vi "GetStringEnumTerminals.vi"(8 "error in (no error)":errorcluster, 9 "WireTerminal":refnum<vi>, 11 "Terms[]":refnum<vi>[](array[refnum])) -> (0 "error out":errorcluster, 3 "Array":refnum<vi>[](array[refnum]))   [LabVIEW 2020, in "Scripting.lvclass"]
uses:
  Scripting.lvclass
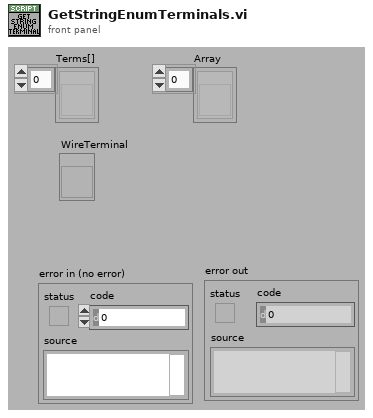
[diagram p1: front panel]
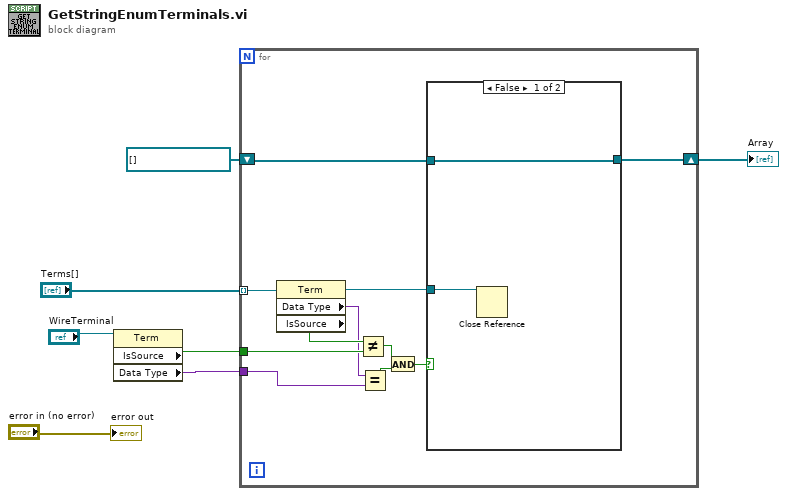
[diagram p0: block diagram]
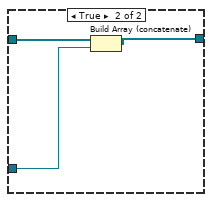
[diagram p2: hidden frame]
diagram:
  n1 = property class="Term"(reference="WireTerminal") -> ("IsSource"=w3:bool, "Data Type"=w2:variant)  [unwired: 1 in, 2 out]
  n2 = for {
    tunnel: "Terms[]" -> [w18] mode=indexing
    tunnel: w3 -> [w16]
    shift-right: [w13] -> w5
    shift-left: refnum<vi>[] [] -> [w15]
    tunnel: w2 -> [w11]
    n3 = property class="Term"(reference=w18) -> (reference out=w14:refnum<vi>, "Data Type"=w12:variant, "IsSource"=w17:bool)  [unwired: 1 in, 1 out]
    n4 = Not Equal?(x=w17, y=w16) -> (x != y?=w9:bool)
    n5 = Equal?(x=w12, y=w11) -> (x = y?=w10:bool)
    n6 = And(x=w9, y=w10) -> (x .and. y?=w8:bool)
    n7 = case shown="False" w8 {
      tunnel: w15 -> [w20 w23]
      tunnel: w14 -> [w19 w22]
      tunnel: [w20 w21] -> w13
      frame False {
        n8 = Close Reference(reference=w19) -> ()  [unwired: 1 in, 1 out]
      }
      frame True {
        n9 = Build Array (concatenate)(w23, w22) -> (w21:refnum<vi>[])
      }
    }
  }
  "Array" <- w5
  "error out" <- "error in (no error)"
